vi "SW_Load_settings_file.vi"(0 "Researchers list reference in":refnum<vi>, 1 "Password field reference in":refnum<vi>) -> (2 "Config refnum out":T1, 3 "Config file path":path, 4 "Users section name":string, 5 "error out":errorcluster)   [LabVIEW 2016]
uses:
  <vilib>/Utility/config.llb/Config Data RefNum.ctl
  <vilib>/Utility/config.llb/NI_LVConfig.lvlib
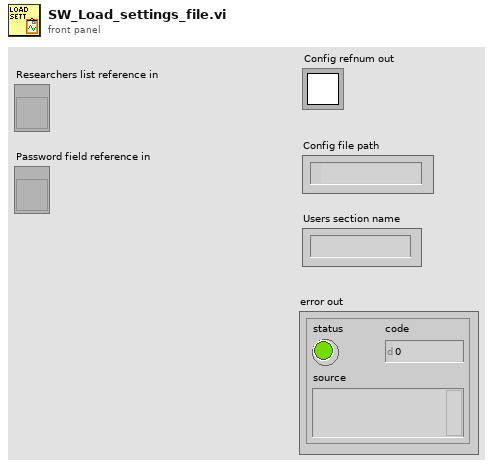
[diagram p1: front panel]
types:
  T1 = typedef "NI_LVConfig.lvlib/Config Data RefNum.ctl" = refnum<k1>
  T2 = enum8{"Enabled", "Disabled", "Disabled and Grayed Out"}
  T3 = enum32{"invalid app kind", "Development System", "Run Time System", "Student Edition", "Embedded LabVIEW", "Evaluation", "Custom"}
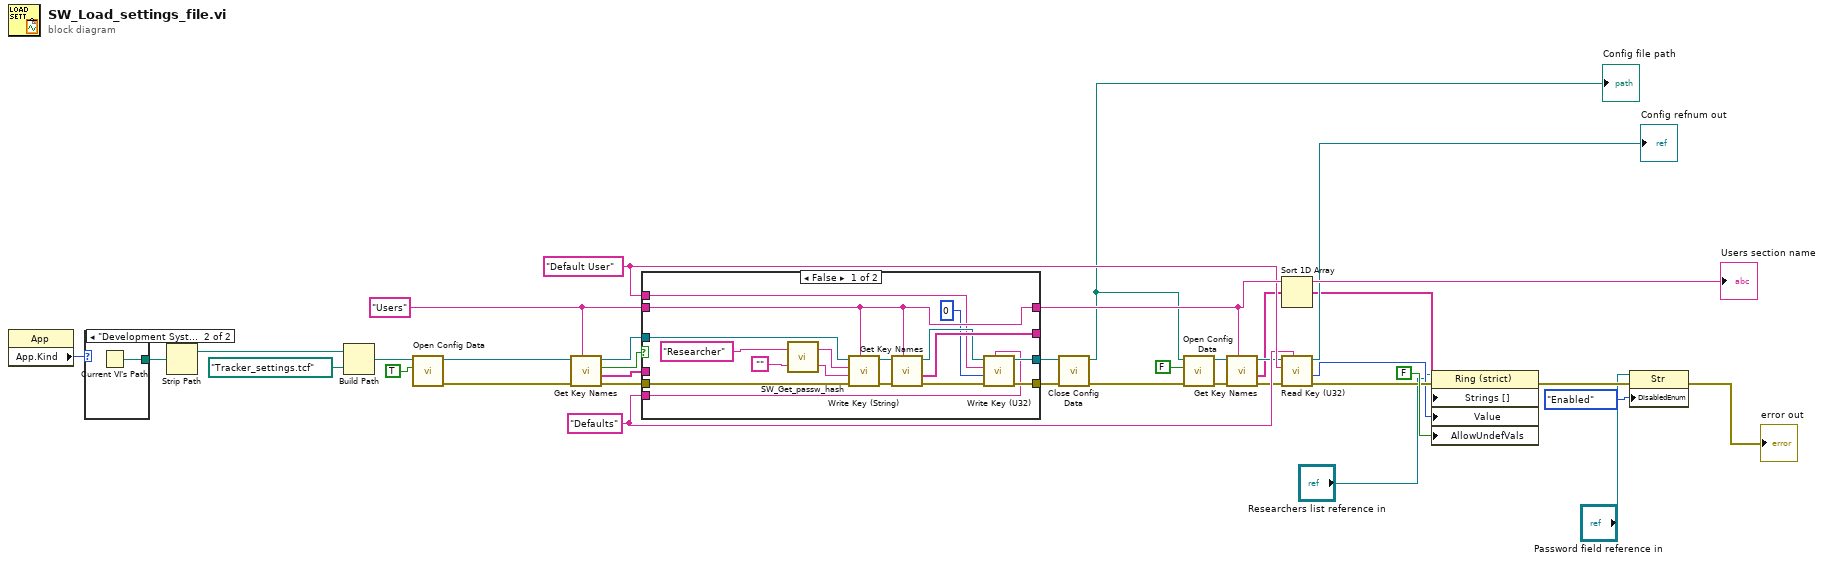
[diagram p0: block diagram]
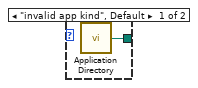
[diagram p3: hidden frame]
diagram:
  w14 = "Users" ("Users section name")
  w27 = "Default User" ("key")
  w26 = "Defaults" ("section")
  n1 = property class="App"() -> ("App.Kind"=w3:T3)  [unwired: 2 in, 2 out]
  n2 = case shown="\"Development System\"" w3 {
    tunnel: [w37 w38] -> w5
    frame "invalid app kind", Default {
      n3 = call <vilib>:"Application Directory.vi"() -> ("Application Directory"=w37:path)
    }
    frame "Development System" {
      n4 = Current VI's Path() -> (path=w38:path)
    }
  }
  n5 = Strip Path(path=w5) -> (stripped path=w6:path)  [unwired: 1 out]
  n6 = Build Path(base path=w6, name or relative path=path "Tracker_settings.tcf") -> (appended path=w7:path)
  n7 = call <vilib>:"Open Config Data.vi"("create file if necessary (T)"=TRUE, "configuration file path"=w7) -> ("error out"=w10:errorcluster, "refnum"=w9:T1)  [unwired: 7 in, 1 out]
  n8 = call <vilib>:"Get Key Names.vi"("section"=w14, "error in (no error)"=w10, "refnum"=w9) -> ("error out"=w12:errorcluster, "key names"=w15:string[], "section exists?"=w11:bool, "refnum out"=w13:T1)  [unwired: 5 in]
  n9 = case shown="False" w11 {
    tunnel: w12 -> [w52 w59]
    tunnel: w13 -> [w53 w58]
    tunnel: w14 -> [w49 w56]
    tunnel: [w43 w58] -> w16
    tunnel: [w44 w59] -> w17
    tunnel: [w54 w57] -> _
    tunnel: w15 -> [_ w57]
    tunnel: [w49 w56] -> w36
    tunnel: w26 -> [w42 _]
    tunnel: w27 -> [w41 _]
    frame False {
      n10 = call "SW_Get_passw_hash.vi"("Password"="" ("string"), "Username"="Researcher" ("string")) -> ("Password hash"=w47:string, "Username"=w48:string)
      n11 = call <vilib>:"Write Key (String).vi"("section"=w49, "error in (no error)"=w52, "value"=w47, "key"=w48, "refnum"=w53) -> ("error out"=w51:errorcluster, "refnum out"=w50:T1)  [unwired: 4 in, 1 out]
      n12 = call <vilib>:"Get Key Names.vi"("section"=w49, "error in (no error)"=w51, "refnum"=w50) -> ("error out"=w45:errorcluster, "key names"=w54:string[], "refnum out"=w46:T1)  [unwired: 5 in, 1 out]
      n13 = call <vilib>:"Write Key (U32).vi"("section"=w42, "error in (no error)"=w45, "value"=u32 0, "key"=w41, "refnum"=w46) -> ("error out"=w44:errorcluster, "refnum out"=w43:T1)  [unwired: 4 in, 1 out]
    }
    frame True {
    }
  }
  "Users section name" <- w36
  n14 = call <vilib>:"Close Config Data.vi"("error in (no error)"=w17, "refnum"=w16) -> ("error out"=w18:errorcluster, "file path"=w19:path)  [unwired: 8 in]
  "Config file path" <- w19
  n15 = call <vilib>:"Open Config Data.vi"("error in (no error)"=w18, "create file if necessary (T)"=FALSE, "configuration file path"=w19) -> ("error out"=w21:errorcluster, "refnum"=w22:T1)  [unwired: 6 in, 1 out]
  n16 = call <vilib>:"Get Key Names.vi"("section"=w36, "error in (no error)"=w21, "refnum"=w22) -> ("error out"=w25:errorcluster, "key names"=w23:string[], "refnum out"=w24:T1)  [unwired: 5 in, 1 out]
  n17 = Sort 1D Array(array=w23) -> (sorted array=w28:string[])
  n18 = call <vilib>:"Read Key (U32).vi"("section"=w26, "error in (no error)"=w25, "key"=w27, "refnum"=w24) -> ("error out"=w30:errorcluster, "value"=w29:u32, "refnum out"=→"Config refnum out":T1)  [unwired: 4 in, 1 out]
  n19 = property on="Property Node" class="Ring (strict)"(reference="Researchers list reference in", error in=w30, "Strings []"=w28, "Value"=w29, "AllowUndefVals"=FALSE ("Allow Undefined Strings")) -> (error out=w32:errorcluster)  [unwired: 1 out]
  n20 = property on="Property Node" class="Str"(reference="Password field reference in", error in=w32, "DisabledEnum"=T2."Enabled" ("Disabled")) -> (error out=→"error out":errorcluster)  [unwired: 1 out]
